vi "Read Encoders.vi"() -> (3 "Angles":T1)   [LabVIEW 2018]
uses:
  <vilib>/Rock Robotics/Network Tables/NT Write Number.vi
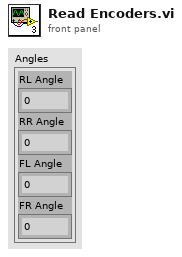
[diagram p1: front panel]
types:
  T1 = cluster{"RL Angle":dbl, "RR Angle":dbl, "FL Angle":dbl, "FR Angle":dbl}
  T2 = typedef "WPI_AnalogChannelDevRef.ctl" = cluster{"DevStatus":errorcluster, "Analog Channel":T3}
  T3 = typedef "FPGA_AIChannel.ctl" = enum8{"AI 0", "AI 1", "AI 2", "AI 3", "AI MXP 0", "AI MXP 1", "AI MXP 2", "AI MXP 3", "Invalid"}
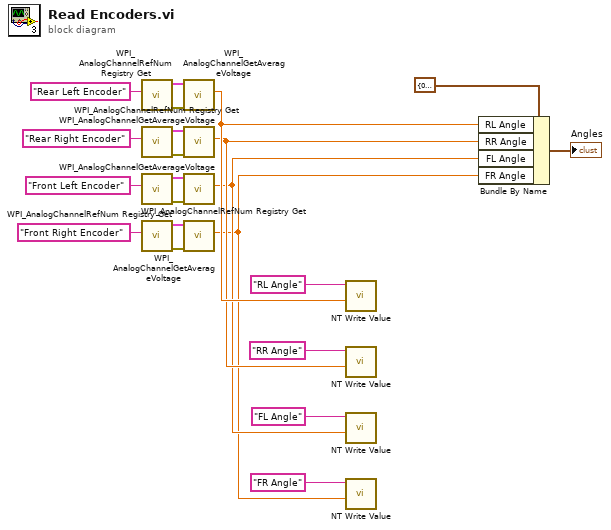
[diagram p0: block diagram]
diagram:
  n1 = call <vilib>:"WPI_AnalogChannelRefNum Registry Get.vi"("refnum name"="Rear Left Encoder") -> ("error out"=w22:errorcluster, "AIDeviceRef"=w21:T2)  [unwired: 9 in]
  n2 = call <vilib>:"WPI_AnalogChannelRefNum Registry Get.vi"("refnum name"="Rear Right Encoder") -> ("error out"=w19:errorcluster, "AIDeviceRef"=w18:T2)  [unwired: 9 in]
  n3 = call <vilib>:"WPI_AnalogChannelRefNum Registry Get.vi"("refnum name"="Front Left Encoder") -> ("error out"=w16:errorcluster, "AIDeviceRef"=w15:T2)  [unwired: 9 in]
  n4 = call <vilib>:"WPI_AnalogChannelRefNum Registry Get.vi"("refnum name"="Front Right Encoder") -> ("error out"=w13:errorcluster, "AIDeviceRef"=w12:T2)  [unwired: 9 in]
  n5 = call <vilib>:"WPI_AnalogChannelGetAverageVoltage.vi"("error in (no error)"=w22, "AIDeviceRef"=w21) -> ("Voltage"=w9:dbl)  [unwired: 7 in, 2 out]
  n6 = call <vilib>:"WPI_AnalogChannelGetAverageVoltage.vi"("error in (no error)"=w19, "AIDeviceRef"=w18) -> ("Voltage"=w8:dbl)  [unwired: 7 in, 2 out]
  n7 = call <vilib>:"WPI_AnalogChannelGetAverageVoltage.vi"("error in (no error)"=w16, "AIDeviceRef"=w15) -> ("Voltage"=w7:dbl)  [unwired: 7 in, 2 out]
  n8 = call <vilib>:"WPI_AnalogChannelGetAverageVoltage.vi"("error in (no error)"=w13, "AIDeviceRef"=w12) -> ("Voltage"=w6:dbl)  [unwired: 7 in, 2 out]
  n9 = call-poly <vilib>:"NT Write Value.vi"("Numeric"=w9, "Name"="RL Angle") -> ()  [unwired: 9 in, 1 out]
  n10 = call-poly <vilib>:"NT Write Value.vi"("Numeric"=w8, "Name"="RR Angle") -> ()  [unwired: 9 in, 1 out]
  n11 = call-poly <vilib>:"NT Write Value.vi"("Numeric"=w7, "Name"="FL Angle") -> ()  [unwired: 9 in, 1 out]
  n12 = call-poly <vilib>:"NT Write Value.vi"("Numeric"=w6, "Name"="FR Angle") -> ()  [unwired: 9 in, 1 out]
  n13 = Bundle By Name(cluster=T1 {"RL Angle"=0.0, "RR Angle"=0.0, "FL Angle"=0.0, "FR Angle"=0.0}, "RL Angle"=w9, "RR Angle"=w8, "FL Angle"=w7, "FR Angle"=w6) -> (→"Angles":T1)
